vi "Set DB.vi"(8 "error in (no error)":errorcluster, 10 "Database":refnum<class "Database Interface.lvclass">, 11 "Column in":refnum<class "Column.lvclass">) -> (0 "error out":errorcluster, 3 "Column out":refnum<class "Column.lvclass">)   [LabVIEW 2020, in "Basic Columns.lvlib" / "Column.lvclass"]
uses:
  Column.lvclass
  Database Interfaces/Database Interface Class/Database Interface.lvclass
  Column.lvclass/Column.ctl
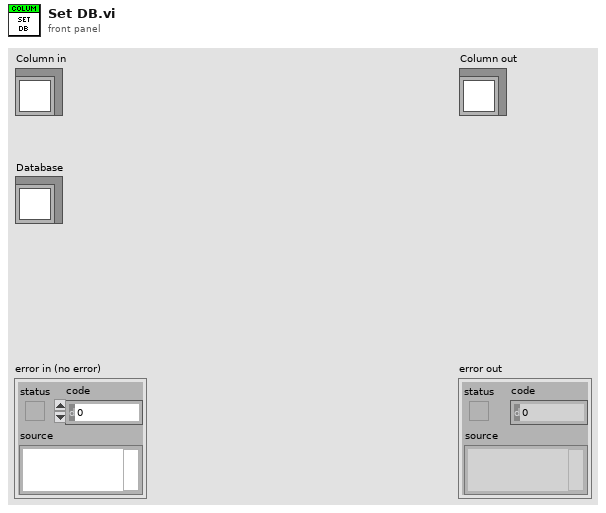
[diagram p1: front panel]
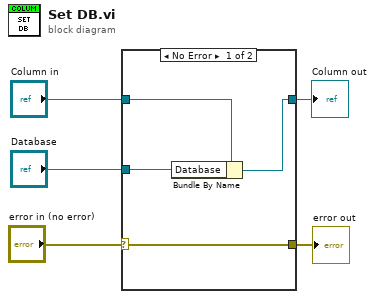
[diagram p0: block diagram]
diagram:
  n1 = case shown="No Error" "error in (no error)" {
    selector: "error in (no error)" -> [w9 w10]
    tunnel: [w9 w10] -> w4
    tunnel: "Column in" -> [w7 w11]
    tunnel: [w6 w11] -> w2
    tunnel: "Database" -> [w8 _]
    frame No Error {
      n2 = Bundle By Name(cluster=w7, "Database"=w8) -> (w6:refnum<class "Column.lvclass">)
    }
    frame Error {
    }
  }
  "error out" <- w4
  "Column out" <- w2
